vi "Enter Password.vi"() -> (0 "Password 2":string)   [LabVIEW 2015, in "Control-Client.lvclass"]
uses:
  Control-Client.lvclass
panel:
  in  "Password":string
  in  "Stop":bool
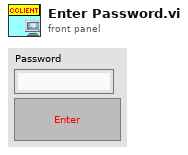
[diagram p1: front panel]
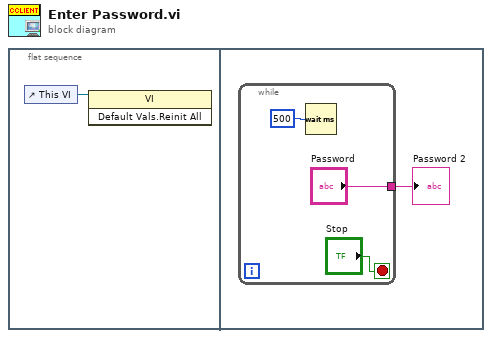
[diagram p0: block diagram]
diagram:
  n1 = flat-sequence {
    frame #0 {
      n2 = control-ref of="This VI"() -> (w1:refnum<vi>)
      n3 = invoke class="VI" method="Default Vals.Reinit All"(reference=w1) -> ()  [unwired: 2 in, 3 out]
    }
    frame #1 {
      n4 = while {
        tunnel: ["Password"] -> w2
        stop <- "Stop" stop-if-true
        n5 = Wait (ms)(milliseconds to wait=u32 500) -> ()  [unwired: 1 out]
      }
      "Password 2" <- w2
    }
  }
